vi "信号光谱3-拟合优化版本.vi"() -> ()   [LabVIEW 2018]
uses:
  <vilib>/Utility/file.llb/Write Delimited Spreadsheet (DBL).vi
  <vilib>/Analysis/NI_AALBase.lvlib
  <vilib>/ptbypt/NI_PtbyPt.lvlib
panel:
  in  "格式字符串":string
  in  "分隔符(Tab)":string
  in  "端口":u16
  in  "地址":string
  out "正在测量":bool
  in  "滤波阈值":dbl=1500.0 format="%#_13g"
  out "best fit":dbl[][](graph) caption="最佳拟合"
  out "范围内？":bool[](array[boolean])
  out "w":dbl
  out "xc":dbl
  out "拟合参数":dbl[](array[numeric])
  out "最终存储路径":path
  in  "停止程序":bool
  in  "上升下降沿/s":dbl format="%.2p"
  in  "延时/s":dbl format="%.2p"
  in  "占空比/%":dbl=3.0 format="%.2p"
  in  "高电平/V":dbl=4.0 format="%.2p"
  in  "频率/Hz":dbl=100.0 format="%.3p"
  in  "低电平/V":dbl min=0.0 max=5.0 format="%.2p"
  out "configure error out":errorcluster
  in  "设置参数":bool
  out "output control error  4":errorcluster
  in  "低电平持续输出":bool
  in  "Output 1":bool
  out "output control error  5":errorcluster
  in  "脉冲作用时间/s":dbl=1.0
  in  "测量高电平/V":dbl=4.0
  out "output control error  2":errorcluster
  in  "测量次数":i32=1
  in  "开始测量":bool
  in  "上升下降沿":i32(ring)=1 items=["上升沿", "下降沿"]
  in  "channel输出口":i32(ring) items=["Channel 1", "Channel 2"]
  in  "输出信号波形":u16(ring) items=["Pulse"]
  out "output control error  3":errorcluster
  out "Output":bool
  in  "VISA 信号发生器":refnum<visa-resource-name>="USB0::0x1AB1::0x0641::DG4E192200870::INSTR"
  out "Spectrum":cluster{"Y":dbl[], "Y":dbl[]}[](graph)
  in  "计数器":dbl=720.0
  out "波长范围":dbl[](array[numeric])
  in  "选项卡控件":enum32{"IHR 550", "CCD"}(tab)
  in  "Move To\nTarget Positions":bool
  out "Current UniqueID":string="Mono4"
  in  "Mono ID":string(combo)="Mono1"
  in  "Connect":bool
  out "Initialized JY":bool=TRUE
  in  "Force\nInitialization":bool
  in  "Target Grating":string(combo)="2"
  out "Current Description":string="1" caption="Description"
  out "Grating Index":i32=1
  out "Current Grating":dbl=1200.0
  out "Units":string="nm"
  out "Current WL":dbl=897.9988
  out "Exit Mirror\nPosition":i32(ring)=2 items=["EntranceMirror", "ExitMirror", "Front", "Side"]
  out "Entrance Mirror\nPosition":i32(ring)=2 items=["EntranceMirror", "ExitMirror", "Front", "Side"]
  out "Units 2":string="mm"
  out "Front Entrance":dbl
  in  "Target WL":dbl=2670.0
  in  "Exit Mirror":u16(ring)=3 caption="Target Position Exit Mirror" items=["Front"=2, "Side"=3]
  in  "Entrance Mirror":u16(ring)=2 caption="Target Position\nEntrance Mirror" items=["Front"=2, "Side"=3]
  in  "Target\nFront Entrance":dbl=1.0
  in  "Commande tab":T1(tab)
  in  "Area Number to Display":i32
  in  "Reformat":bool
  in  "GAIN":u16(ring)=2 caption="Device Name" items=["High Light", "Best Dynamic Range", "High Sensitivity"]
  in  "ADC":u16(ring) caption="Device Name" items=["20 kHz       ", " 1 MHz       ", " 1 MHz Ultra "]
  in  "Number of Areas :":u16=1 min=1 step=1
  in  "Integration time (ms) :":i16=5000
  out "Uniques ID":u16(ring) items=["CCD1", "CCD2"]
  in  "Device Name":u16(ring) items=["Synapse CCD (Lateral)", "Synapse_IGA (Axial)"]
  in  "Signal type :":enum16{"TTL Rising Edge", "TTL Falling Edge"}(ring)=enum."TTL Falling Edge"
  in  "Trigger Type :":u16(ring) items=["On Start"=1, "Per Acquisition"=2]
  in  "trigSigTypeString":string
  in  "trigEventString":string
  in  "Enable InputTriggers :":bool
  in  "Number of Cleans":i32=1
  in  "MultiAcqShutterMode":i32(ring)=3 items=["Open For All Spectra"=1, "Open for Each Spectrum"=3]
  in  "Accumulations:":u16=10 min=1 step=1
  in  "Multi Accumulation mode:":bool
  out "Y Pixels:":i32=256
  out "DataSize":i32=1024
  out "X Pixels:":i32=1024
  out "Firmware\nVersion":string="V1.20 CCD_4000"
  out "initialized ?":bool=TRUE
  in  "Continuous":bool
  in  "CCD Busy":bool
  out "indicator":string="Ready !"
  in  "initialize":bool
  in  "ShutterOpen":bool=TRUE caption="Shutter enable"
  in  "Acquire":bool
  in  "Temperature":bool
  in  "Setup":bool
  in  "起始波长":dbl=2406.79
  in  "终止波长":dbl=2919.91
  out "Acq Time(ms)":u32=3401
  in  "Save Backlight":bool
  in  "cut backlight":bool
  out "backlight":bool=TRUE
  in  "Close":bool=TRUE
  out "JYCCDLib.IJYCCDReqd":refnum<k7>
  out "areas :":i32[][](array[numeric])=[[1], [1], [1], [1024], [256], [1], [256]]
  in  "Constante de condition\n(Voir l'aide contextuelle)":bool
  out "temp graph":dbl(graph)=-134.538067
  out "ADC Number":i32[](array[numeric])=[0, 1, 2, 3, 4]
  out "Gain Number":i32[](array[numeric])=[10, 11, 12, 13, 8, 2]
  out "trigAddress":i32
  out "Data":i32[][](graph)
  out "error out":errorcluster
  out "Gratings":dbl[](array[numeric])=[1200.0, 300.0]
  out "Backlight":i32[][](graph)
  out "data 2":i32[][](graph)
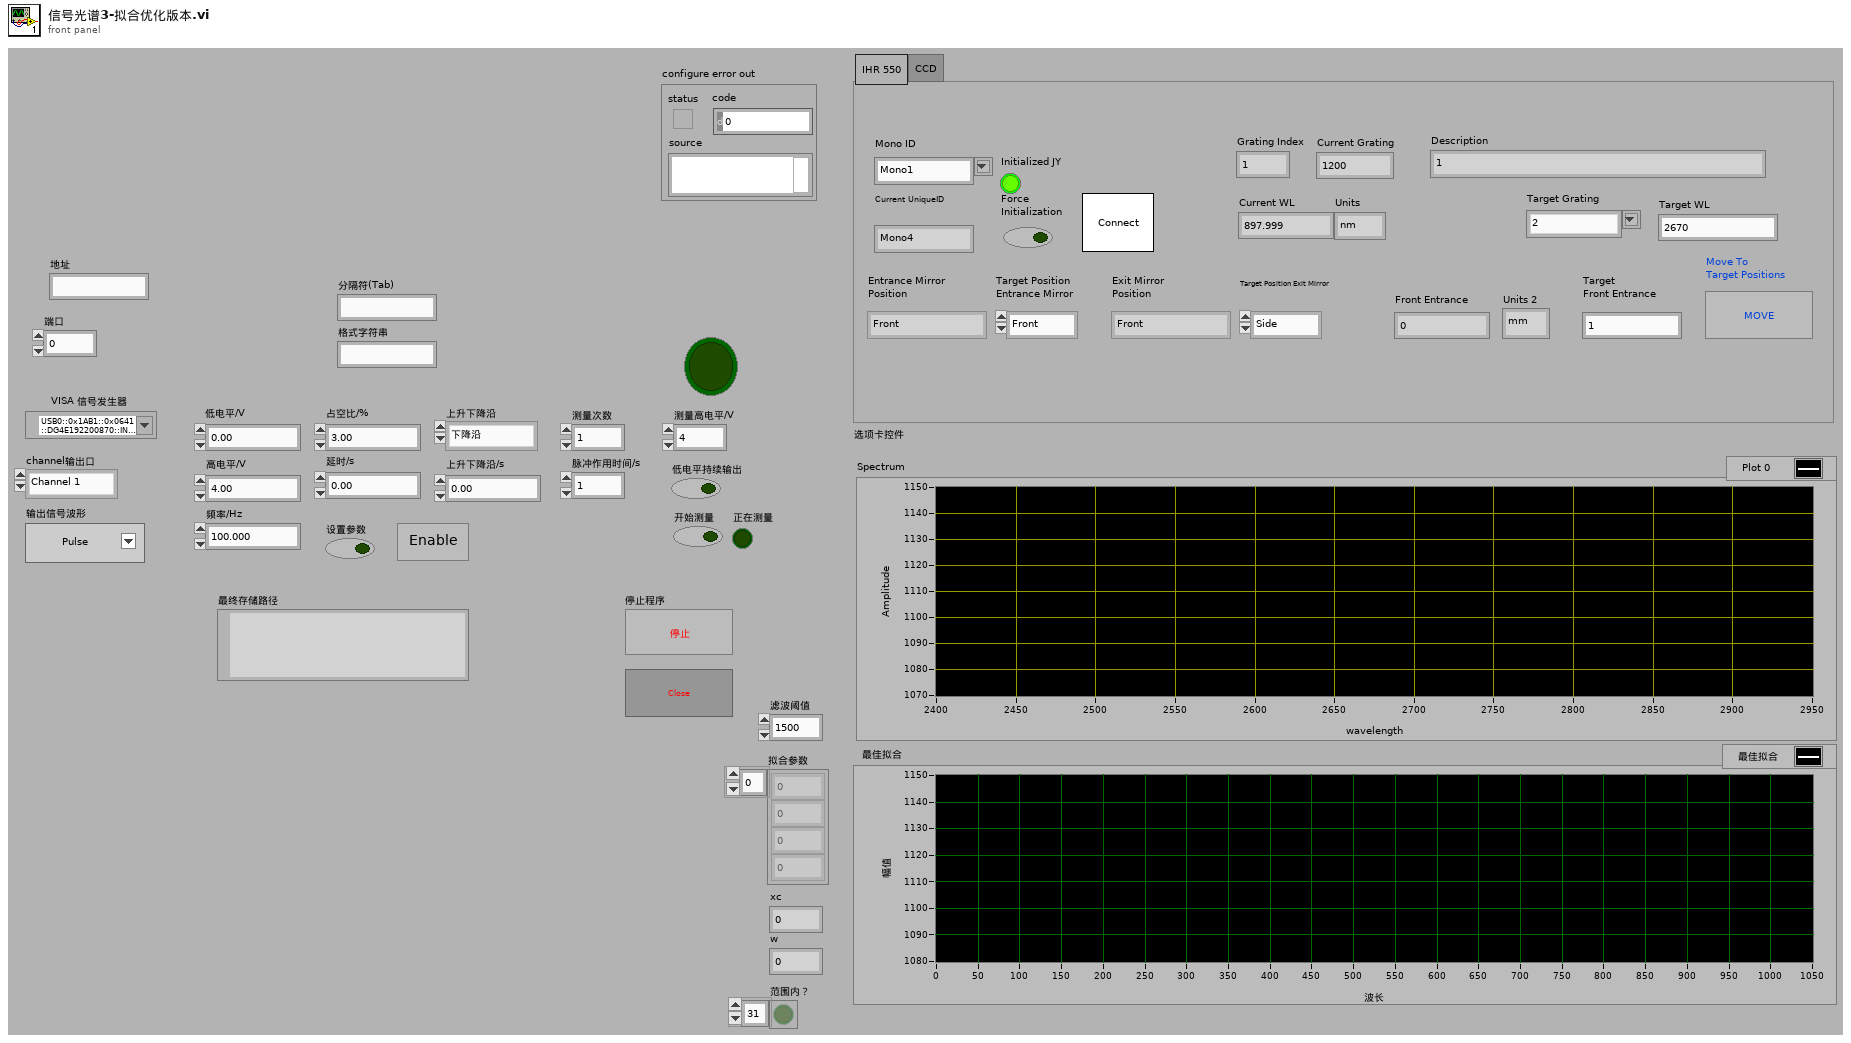
[diagram p1: front panel]
types:
  T1 = enum32{"Settings", "Trigger In", "Multi-Accu.", "Infos"}
  T2 = enum8{"Enabled", "Disabled", "Disabled and Grayed Out"}
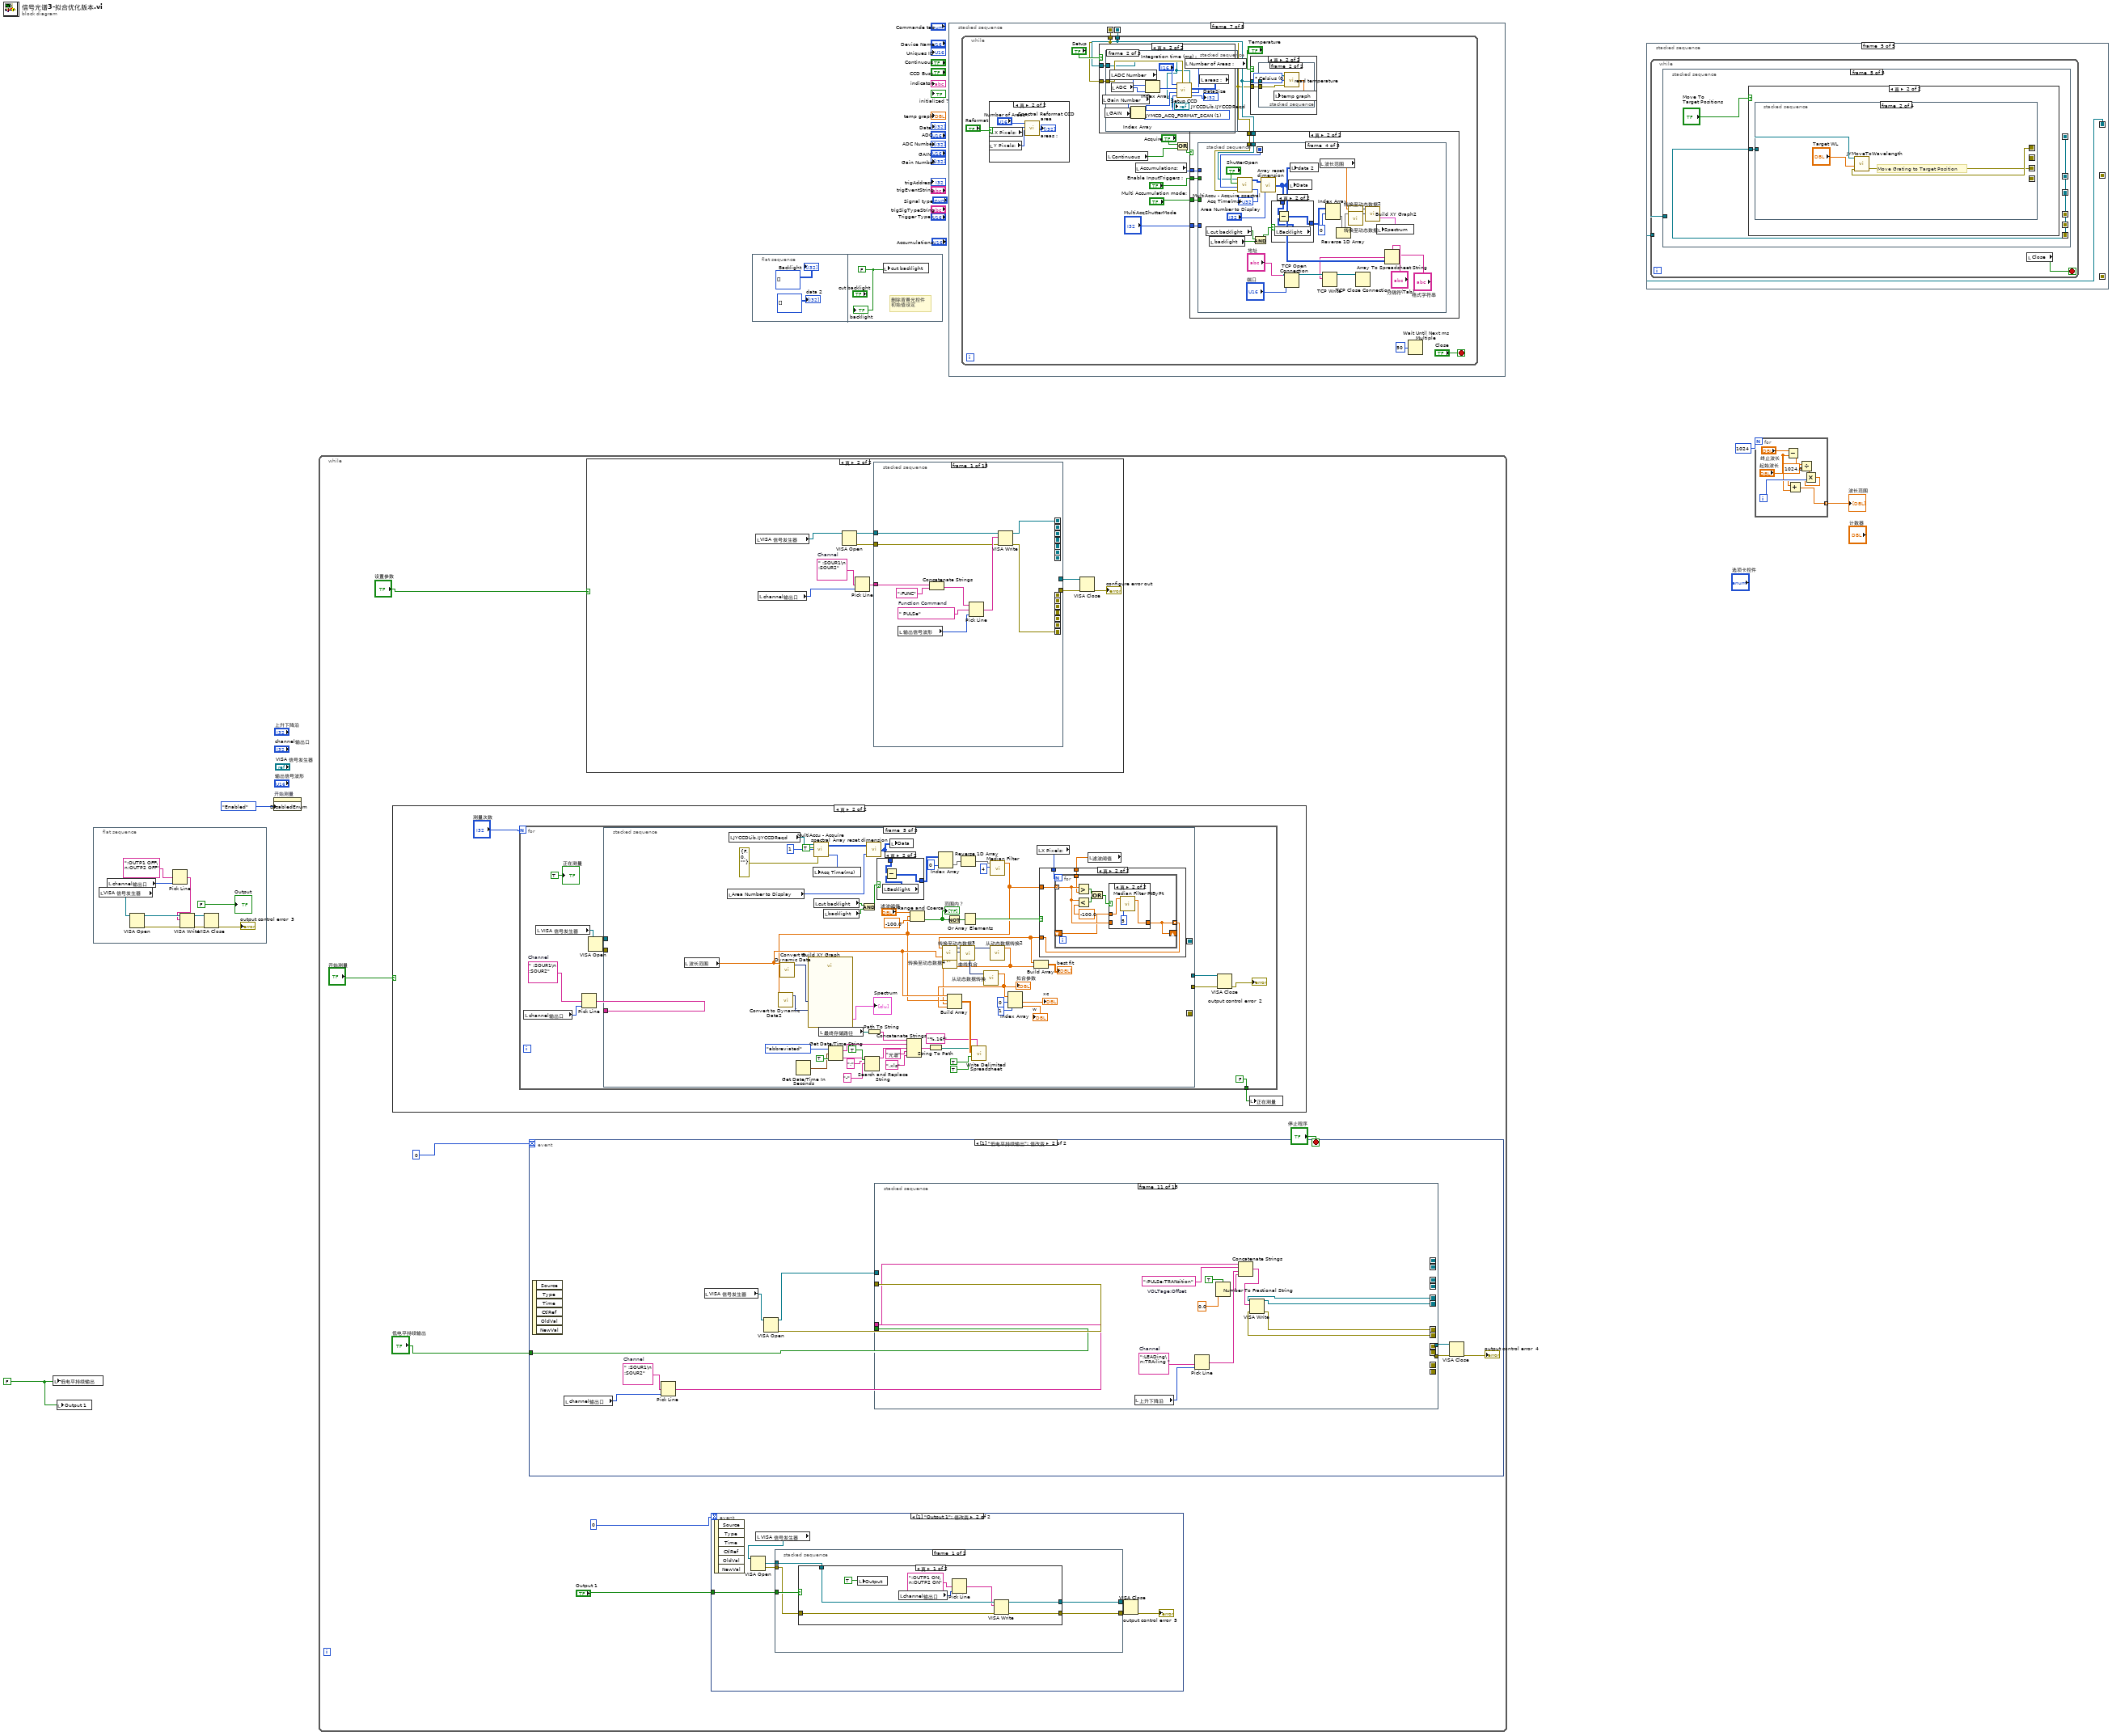
[diagram p0: block diagram]
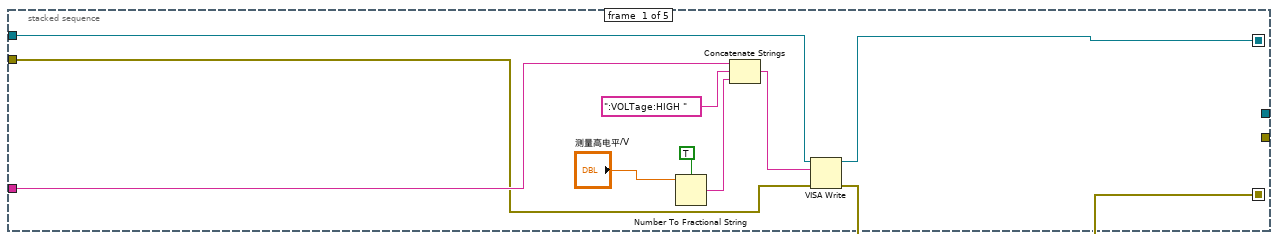
[diagram p3: hidden frame]
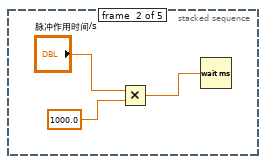
[diagram p4: hidden frame]
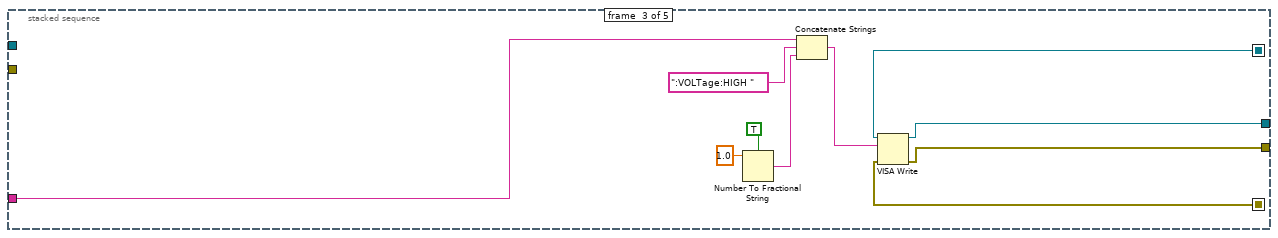
[diagram p5: hidden frame]
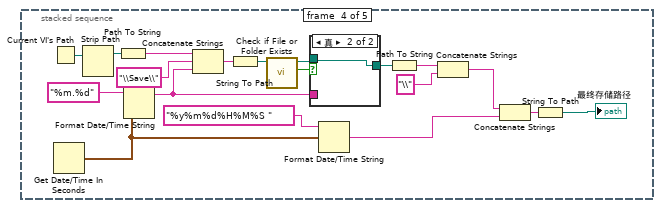
[diagram p6: hidden frame]
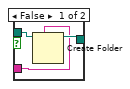
[diagram p7: hidden frame]
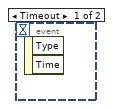
[diagram p11: hidden frame]
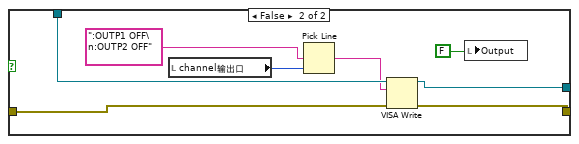
[diagram p12: hidden frame]
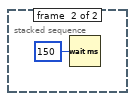
[diagram p13: hidden frame]
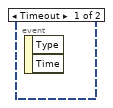
[diagram p14: hidden frame]
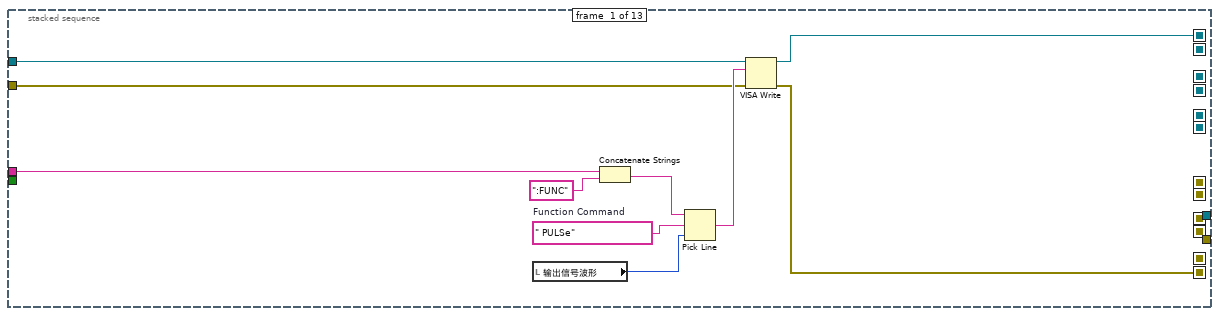
[diagram p15: hidden frame]
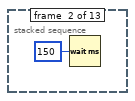
[diagram p16: hidden frame]
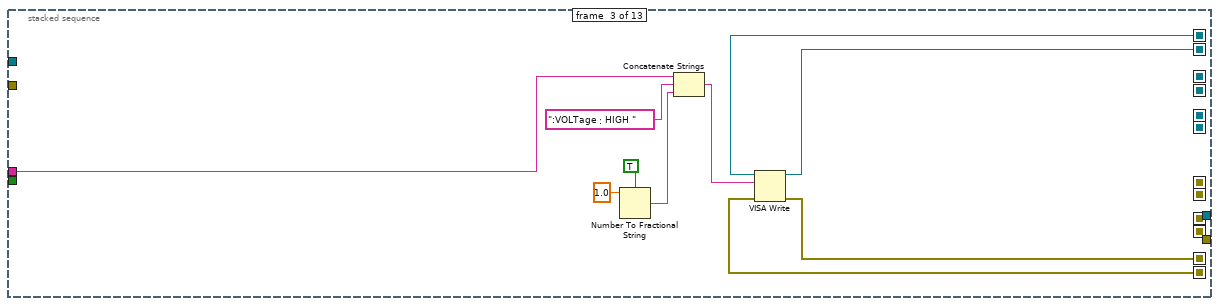
[diagram p17: hidden frame]
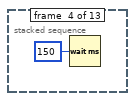
[diagram p18: hidden frame]
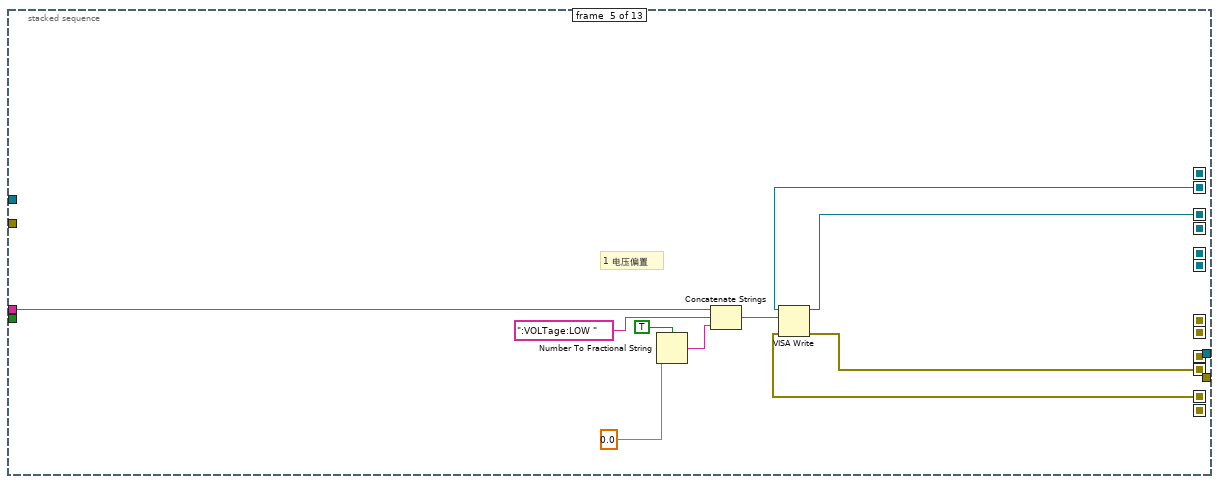
[diagram p19: hidden frame]
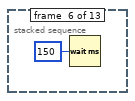
[diagram p20: hidden frame]
diagram:
  w1 = FALSE
  n1 = local write "低电平持续输出"(w1) -> ()
  n2 = local write "Output 1"(w1) -> ()
  n3 = flat-sequence {
    frame #0 {
      n4 = local read "VISA 信号发生器"() -> (w8:refnum<visa-resource-name>)
      n5 = local read "channel输出口"() -> (w6:i32)
      n6 = VISA Open(VISA resource name=w8) -> (VISA resource name=w14:refnum<visa-resource-name>, error out=w13:errorcluster)  [unwired: 4 in]
      n7 = Pick Line(multi-line string=":OUTP1 OFF\n:OUTP2 OFF" ("write buffer"), line index=w6) -> (output string=w5:string)  [unwired: 1 in]
      n8 = VISA Write(VISA resource name=w14, write buffer=w5, error in (no error)=w13) -> (VISA resource name out=w11:refnum<visa-resource-name>, error out=w10:errorcluster)  [unwired: 1 out]
      n9 = VISA Close(VISA resource name=w11, error in (no error)=w10) -> (error out=→"output control error  3":errorcluster)
      "Output" <- FALSE ("布尔")
    }
  }
  n10 = property on="开始测量" class="Bool"("DisabledEnum"=T2."Enabled" ("禁用")) -> ()  [unwired: 2 in, 2 out]
  n11 = while {
    stop <- "停止程序" stop-if-true
    n12 = case shown="真" "开始测量" {
      frame False {
      }
      frame True {
        n13 = for {
          N: "测量次数" -> [_]
          tunnel: [FALSE] -> w22
          w27 = " :SOUR1\n :SOUR2"  # Channel
          n14 = local read "channel输出口"() -> (w28:i32)
          n15 = local read "VISA 信号发生器"() -> (w34:refnum<visa-resource-name>)
          n16 = Pick Line(multi-line string=w27, line index=w28) -> (output string=w26:string)  [unwired: 1 in]
          n17 = VISA Open(VISA resource name=w34) -> (VISA resource name=w33:refnum<visa-resource-name>, error out=w32:errorcluster)  [unwired: 4 in]
          n18 = stacked-sequence {
            seq-local: [w37 _ _ _ _] -> [_ _ w50 _ _]
            seq-local: [w36 _ _ _ _] -> [_ _ w49 _ _]
            tunnel: w33 -> [w39 _ _ _ _]
            tunnel: w32 -> [w38 _ _ _ _]
            tunnel: [_ _ w52 _ _] -> w31
            tunnel: [_ _ w51 _ _] -> w30
            tunnel: w26 -> [w40 _ w48 _ _]
            frame #0 {
              n19 = Number To Fractional String(use system decimal point (T)=TRUE ("使用系统小数点(T)"), number="测量高电平/V") -> (F-format string=w42:string)  [unwired: 2 in]
              n20 = Concatenate Strings ("连接字符串")(w40, ":VOLTage:HIGH ", w42) -> (w41:string)
              n21 = VISA Write(VISA resource name=w39, write buffer=w41, error in (no error)=w38) -> (VISA resource name out=w37:refnum<visa-resource-name>, error out=w36:errorcluster)  [unwired: 1 out]
            }
            frame #1 {
              n22 = Multiply(x="脉冲作用时间/s", y=1000.0) -> (x*y=w45:dbl)
              n23 = Wait (ms)(milliseconds to wait=w45) -> ()  [unwired: 1 out]
            }
            frame #2 {
              n24 = Number To Fractional String(use system decimal point (T)=TRUE ("使用系统小数点(T)"), number=1.0 ("数字")) -> (F-format string=w55:string)  [unwired: 2 in]
              n25 = Concatenate Strings ("连接字符串")(w48, ":VOLTage:HIGH ", w55) -> (w54:string)
              n26 = VISA Write(VISA resource name=w50, write buffer=w54, error in (no error)=w49) -> (VISA resource name out=w52:refnum<visa-resource-name>, error out=w51:errorcluster)  [unwired: 1 out]
            }
            frame #3 {
              n27 = Current VI's Path() -> (path=w63:path)
              n28 = Get Date/Time In Seconds() -> (seconds since 1Jan1904=w65:timestamp)
              n29 = Strip Path(path=w63) -> (stripped path=w64:path)  [unwired: 1 out]
              n30 = Path To String(path=w64) -> (string=w66:string)
              n31 = Format Date/Time String(time format string (%c)="%m.%d" ("时间格式字符串(%c)"), seconds (now)=w65) -> (date/time string=w72:string)  [unwired: 1 in]
              n32 = Concatenate Strings(w66, "\\Save\\" ("字符串"), w72) -> (w67:string)
              n33 = String To Path(string=w67) -> (path=w68:path)
              n34 = call <vilib>:"Check if File or Folder Exists.vi"("path"=w68) -> ("file or folder exists?"=w69:bool, "dup path"=w71:path)  [unwired: 8 in, 1 out]
              n35 = case shown="真" w69 {
                tunnel: [w79 w80] -> w70
                tunnel: w71 -> [w78 w80]
                tunnel: w72 -> [w77 _]
                frame False {
                  n36 = Create Folder(prompt (Create Folder)=w77, path (use dialog)=w78) -> (created path=w79:path)  [unwired: 1 in, 2 out]
                }
                frame True {
                }
              }
              n37 = Format Date/Time String(time format string (%c)="%y%m%d%H%M%S " ("时间格式字符串(%c)"), seconds (now)=w65) -> (date/time string=w75:string)  [unwired: 1 in]
              n38 = Path To String(path=w70) -> (string=w73:string)
              n39 = Concatenate Strings(w73, "\\" ("字符串")) -> (w74:string)
              n40 = Concatenate Strings(w74, w75) -> (w62:string)
              n41 = String To Path(string=w62) -> (path=→"最终存储路径":path)
            }
            frame #4 {
              n42 = local read "波长范围"() -> (w103:dbl[])
              n43 = local read "Area Number to Display"() -> (w113:i32)
              n44 = local read "JYCCDLib.IJYCCDReqd"() -> (w109:refnum<k7>)
              n45 = call "Convert to Dynamic Data"("Array"=w103) -> ("Dynamic Data Type"=w106:dynamicdata)  [unwired: 3 in]
              n46 = Get Date/Time In Seconds() -> (seconds since 1Jan1904=w122:timestamp)
              n47 = call "MultiAccu - Acquire spectral.vi"("error in"=errorcluster {"status"=FALSE, "code"=0, "source"=""}, "Accumulations:"=u16 1, "ShutterOpen"=TRUE, "JYCCDLib.IJYCCDReqd"=w109) -> ("Acq Time(ms)"=w115:u32, "Array Out"=w114:i32[][][])  [unwired: 1 out]
              n48 = local write "Acq Time(ms)"(w115) -> ()
              n49 = local read "cut backlight"() -> (w94:bool)
              n50 = local read "最终存储路径"() -> (w136:path)
              n51 = local read "backlight"() -> (w92:bool)
              n52 = Get Date/Time String(date format (0)=enum16{"short", "long", "abbreviated"}."abbreviated" ("日期格式(0)"), seconds (now)=w122, want seconds? (F)=TRUE ("需要秒？(F)")) -> (date string=w130:string, time string=w125:string)
              n53 = And(x=w94, y=w92) -> (x .and. y?=w93:bool)
              n54 = Search and Replace String(replace all?=TRUE ("替换全部？(F)"), input string=w125, search string=":" ("搜索字符串"), replace string="-" ("替换字符串(\"\")")) -> (result string=w129:string)  [unwired: 4 in, 3 out]
              n55 = call "Array reset dimension.vi"("Area Number"=w113, "Array In"=w114) -> ("Array Out"=w96:i32[][])
              n56 = Path To String(path=w136) -> (string=w119:string)
              n57 = case shown="真" w93 {
                tunnel: [w157 w159] -> w95
                tunnel: w96 -> [w157 w158]
                frame False {
                }
                frame True {
                  n58 = local read "Backlight"() -> (w160:i32[][])
                  n59 = Subtract(x=w158, y=w160) -> (x-y=w159:i32[][])
                }
              }
              n60 = local write "Data"(w96) -> ()
              n61 = Concatenate Strings(w119, w130, w129, "光谱" ("字符串"), ".xls" ("字符串")) -> (w134:string)
              n62 = String To Path(string=w134) -> (path=w135:path)
              n63 = Index Array(array=w95, index (row)=0 ("索引 (行)")) -> (element=w137:i32[])  [unwired: 1 in]
              n64 = call "转换至动态数据4"("Array"=w103) -> ("Dynamic Data Type"=w102:dynamicdata)  [unwired: 3 in]
              n65 = Reverse 1D Array(array=w137) -> (reversed array=w138:i32[])
              n66 = call <vilib>:"Median Filter.vi"("left rank"=4, "X"=w138) -> ("Filtered X"=w87:dbl[])  [unwired: 8 in, 1 out]
              n67 = call "Convert to Dynamic Data2"("Array"=w87) -> ("Dynamic Data Type"=w105:dynamicdata)  [unwired: 3 in]
              n68 = call "Build XY Graph"("Y Input"=w105, "X Input"=w106) -> ("XY Graph"=→"Spectrum":cluster{"Y":dbl[], "Y":dbl[]}[])  [unwired: 8 in, 1 out]
              n69 = In Range and Coerce(upper limit="滤波阈值", x=w87, lower limit=-100.0) -> (In Range?=w86:bool[])  [unwired: 1 out]
              "范围内？" <- w86
              n70 = Not(x=w86) -> (.not. x?=w85:bool[])
              n71 = Or Array Elements(Boolean array=w85) -> (logical OR=w89:bool)
              n72 = local read "X Pixels:"() -> (w88:i32)
              n73 = local read "滤波阈值"() -> (w81:dbl)
              n74 = case shown="真" w89 {
                tunnel: w88 -> [_ w144]
                tunnel: w87 -> [w140 w143]
                tunnel: [w140 w142] -> w84
                tunnel: w81 -> [_ w141]
                frame False {
                }
                frame True {
                  n75 = for {
                    N: w144 -> [_]
                    tunnel: w143 -> [w148] mode=indexing
                    tunnel: [w147] -> w142 mode=indexing
                    shift-right: [w147] -> _
                    shift-left: _ -> [w146]
                    tunnel: w141 -> [w145]
                    n76 = Greater?(x=w148, y=w145) -> (0:w150:bool)
                    n77 = Less?(x=w148, y=-100.0) -> (x < y?=w151:bool)
                    n78 = Or(x=w150, y=w151) -> (x .or. y?=w149:bool)
                    n79 = case shown="真" w149 {
                      tunnel: w148 -> [w153 _]
                      tunnel: [w153 w155] -> w147
                      tunnel: w146 -> [_ w156]
                      frame False {
                      }
                      frame True {
                        n80 = call <vilib>:"Median Filter PtByPt.vi"("rank"=5, "x"=w156) -> ("Filtered x"=w155:dbl)  [unwired: 2 in, 1 out]
                      }
                    }
                  }
                }
              }
              n81 = call "转换至动态数据3"("Array"=w84) -> ("Dynamic Data Type"=w104:dynamicdata)  [unwired: 3 in]
              n82 = call "曲线拟合"("Locations"=w102, "Signals"=w104) -> ("best fit"=w108:dynamicdata, "non-linear coefficients"=w107:dynamicdata)  [unwired: 5 in, 3 out]
              n83 = call "从动态数据转换"("Dynamic Data Type"=w107) -> ("Array"=w99:dbl[])  [unwired: 3 in]
              "拟合参数" <- w99
              n84 = call "从动态数据转换2"("Dynamic Data Type"=w108) -> ("Array"=w83:dbl[])  [unwired: 3 in]
              n85 = Build Array(w103, w87, w83, w99) -> (w139:dbl[][])
              n86 = call-poly <vilib>:"Write Delimited Spreadsheet.vi"("file path (dialog if empty)"=w135, "format (%.3f)"="%.16f", "2D data"=w139, "append to file? (new file:F)"=TRUE ("append to file? (F)"), "transpose? (no:F)"=TRUE ("transpose? (F)")) -> ()  [unwired: 9 in, 2 out]
              n87 = Index Array(array=w99, index #1=0 ("索引"), index #2=1 ("索引")) -> (element #1=→"xc":dbl, element #2=→"w":dbl)
              n88 = Build Array(w84, w83) -> (→"best fit":dbl[][])
            }
          }
          n89 = VISA Close(VISA resource name=w31, error in (no error)=w30) -> (error out=→"output control error  2":errorcluster)
          "正在测量" <- TRUE
        }
        n90 = local write "正在测量"(w22) -> ()
      }
    }
    n91 = event shown="[1] \"低电平持续输出\": 值改变" {
      selector: _ -> [_ _]
      dyn-events: _ -> [_ _]
      timeout: u32 0 ("Time") -> [_ _]
      tunnel: "低电平持续输出" -> [_ w190]
      event Timeout {
        n92 = event-data() -> ()  [unwired: 1 in, 2 out]
      }
      event "低电平持续输出": Value Change {
        w194 = " :SOUR1\n :SOUR2"  # Channel
        n93 = event-data() -> ()  [unwired: 1 in, 6 out]
        n94 = local read "channel输出口"() -> (w195:i32)
        n95 = Pick Line(multi-line string=w194, line index=w195) -> (output string=w193:string)  [unwired: 1 in]
        n96 = local read "VISA 信号发生器"() -> (w198:refnum<visa-resource-name>)
        n97 = VISA Open(VISA resource name=w198) -> (VISA resource name=w197:refnum<visa-resource-name>, error out=w196:errorcluster)  [unwired: 4 in]
        n98 = stacked-sequence {
          seq-local: [w204 _ _ _ _ _ _ _ _ _ _ _ _] -> [_ _ w219 _ _ _ _ _ _ _ _ _ _]
          seq-local: [w203 _ _ _ _ _ _ _ _ _ _ _ _] -> [_ _ w218 _ _ _ _ _ _ _ _ _ _]
          seq-local: [_ _ w217 _ _ _ _ _ _ _ _ _ _] -> [_ _ _ _ w222 _ _ _ _ _ _ _ _]
          seq-local: [_ _ w216 _ _ _ _ _ _ _ _ _ _] -> [_ _ _ _ w223 _ _ _ _ _ _ _ _]
          seq-local: [_ _ _ _ w231 _ _ _ _ _ _ _ _] -> [_ _ _ _ _ _ w242 _ _ _ _ _ _]
          seq-local: [_ _ _ _ w230 _ _ _ _ _ _ _ _] -> [_ _ _ _ _ _ w241 _ _ _ _ _ _]
          seq-local: [_ _ _ _ _ _ w235 _ _ _ _ _ _] -> [_ _ _ _ _ _ _ _ w245 _ _ _ _]
          seq-local: [_ _ _ _ _ _ w234 _ _ _ _ _ _] -> [_ _ _ _ _ _ _ _ w244 _ _ _ _]
          seq-local: [_ _ _ _ _ _ _ _ w248 _ _ _ _] -> [_ _ _ _ _ _ _ _ _ _ w259 _ _]
          seq-local: [_ _ _ _ _ _ _ _ w247 _ _ _ _] -> [_ _ _ _ _ _ _ _ _ _ w258 _ _]
          seq-local: [_ _ _ _ _ _ _ _ _ _ w256 _ _] -> [_ _ _ _ _ _ _ _ _ _ _ _ w273]
          seq-local: [_ _ _ _ _ _ _ _ _ _ w255 _ _] -> [_ _ _ _ _ _ _ _ _ _ _ _ w272]
          tunnel: w197 -> [w209 _ _ _ _ _ _ _ _ _ _ _ _]
          tunnel: w196 -> [w202 _ _ _ _ _ _ _ _ _ _ _ _]
          tunnel: w193 -> [w201 _ w215 _ w228 _ w239 _ w249 _ w262 _ _]
          tunnel: [_ _ _ _ _ _ _ _ _ _ _ _ w271] -> w192
          tunnel: [_ _ _ _ _ _ _ _ _ _ _ _ w269] -> w191
          tunnel: w190 -> [_ _ _ _ _ _ _ _ _ _ _ _ w270]
          frame #0 {
            w206 = " PULSe"  # Function Command
            n99 = local read "输出信号波形"() -> (w200:u16)
            n100 = Concatenate Strings(w201, ":FUNC" ("string (\"\")")) -> (w207:string)
            n101 = Pick Line(string ("")=w207, multi-line string=w206, line index=w200) -> (output string=w205:string)
            n102 = VISA Write(VISA resource name=w209, write buffer=w205, error in (no error)=w202) -> (VISA resource name out=w204:refnum<visa-resource-name>, error out=w203:errorcluster)  [unwired: 1 out]
          }
          frame #1 {
            n103 = Wait (ms)(milliseconds to wait=u32 150) -> ()  [unwired: 1 out]
          }
          frame #2 {
            n104 = Number To Fractional String(use system decimal point (T)=TRUE ("使用系统小数点(T)"), number=1.0 ("数字")) -> (F-format string=w213:string)  [unwired: 2 in]
            n105 = Concatenate Strings ("连接字符串")(w215, ":VOLTage：HIGH ", w213) -> (w212:string)
            n106 = VISA Write(VISA resource name=w219, write buffer=w212, error in (no error)=w218) -> (VISA resource name out=w217:refnum<visa-resource-name>, error out=w216:errorcluster)  [unwired: 1 out]
          }
          frame #3 {
            n107 = Wait (ms)(milliseconds to wait=u32 150) -> ()  [unwired: 1 out]
          }
          frame #4 {
            # "1 电压偏置"
            n108 = Number To Fractional String(use system decimal point (T)=TRUE ("使用系统小数点(T)"), number=0.0 ("数字")) -> (F-format string=w226:string)  [unwired: 2 in]
            n109 = Concatenate Strings(w228, ":VOLTage:LOW ", w226) -> (w227:string)
            n110 = VISA Write(VISA resource name=w222, write buffer=w227, error in (no error)=w223) -> (VISA resource name out=w231:refnum<visa-resource-name>, error out=w230:errorcluster)  [unwired: 1 out]
          }
          frame #5 {
            n111 = Wait (ms)(milliseconds to wait=u32 150) -> ()  [unwired: 1 out]
          }
          frame #6 {
            n112 = local read "channel输出口"() -> (w237:i32)
            n113 = Pick Line(multi-line string=":OUTP1:IMPedance \n:OUTP2:IMPedance " ("write buffer"), line index=w237) -> (output string=w236:string)  [unwired: 1 in]
            n114 = Concatenate Strings ("连接字符串")(w239, w236, "INFINITY") -> (w240:string)
            n115 = VISA Write(VISA resource name=w242, write buffer=w240, error in (no error)=w241) -> (VISA resource name out=w235:refnum<visa-resource-name>, error out=w234:errorcluster)  [unwired: 1 out]
          }
          frame #7 {
            n116 = Wait (ms)(milliseconds to wait=u32 150) -> ()  [unwired: 1 out]
          }
          frame #8 {
            n117 = Number To Fractional String(use system decimal point (T)=TRUE ("使用系统小数点(T)"), number=0.0 ("数字")) -> (F-format string=w252:string)  [unwired: 2 in]
            n118 = Concatenate Strings(w249, ":PULSe:DELay ", w252) -> (w250:string)
            n119 = VISA Write(VISA resource name=w245, write buffer=w250, error in (no error)=w244) -> (VISA resource name out=w248:refnum<visa-resource-name>, error out=w247:errorcluster)  [unwired: 1 out]
          }
          frame #9 {
            n120 = Wait (ms)(milliseconds to wait=u32 150) -> ()  [unwired: 1 out]
          }
          frame #10 {
            w263 = ":LEADing\n:TRAiling "  # Channel
            w267 = ":PULSe:TRANsition"  # VOLTage:Offset
            n121 = local read "上升下降沿"() -> (w264:i32)
            n122 = Pick Line(multi-line string=w263, line index=w264) -> (output string=w260:string)  [unwired: 1 in]
            n123 = Number To Fractional String(use system decimal point (T)=TRUE ("使用系统小数点(T)"), number=0.0 ("数字")) -> (F-format string=w261:string)  [unwired: 2 in]
            n124 = Concatenate Strings(w262, w267, w260, w261) -> (w265:string)
            n125 = VISA Write(VISA resource name=w259, write buffer=w265, error in (no error)=w258) -> (VISA resource name out=w256:refnum<visa-resource-name>, error out=w255:errorcluster)  [unwired: 1 out]
          }
          frame #11 {
            n126 = Wait (ms)(milliseconds to wait=u32 150) -> ()  [unwired: 1 out]
          }
          frame #12 {
            n127 = case shown="假" w270 {
              tunnel: w273 -> [w281 w282]
              tunnel: [w280 w289] -> w269
              tunnel: w272 -> [w279 w287]
              tunnel: [w278 w288] -> w271
              frame True {
                n128 = local write "Output"(TRUE ("布尔")) -> ()
                n129 = local read "channel输出口"() -> (w275:i32)
                n130 = Pick Line(multi-line string=":OUTP1 ON\n:OUTP2 ON" ("write buffer"), line index=w275) -> (output string=w274:string)  [unwired: 1 in]
                n131 = VISA Write(VISA resource name=w281, write buffer=w274, error in (no error)=w279) -> (VISA resource name out=w278:refnum<visa-resource-name>, error out=w280:errorcluster)  [unwired: 1 out]
              }
              frame False {
                n132 = local read "channel输出口"() -> (w284:i32)
                n133 = Pick Line(multi-line string=":OUTP1 OFF\n:OUTP2 OFF" ("write buffer"), line index=w284) -> (output string=w283:string)  [unwired: 1 in]
                n134 = VISA Write(VISA resource name=w282, write buffer=w283, error in (no error)=w287) -> (VISA resource name out=w288:refnum<visa-resource-name>, error out=w289:errorcluster)  [unwired: 1 out]
                n135 = local write "Output"(FALSE ("布尔")) -> ()
              }
            }
          }
        }
        n136 = VISA Close(VISA resource name=w192, error in (no error)=w191) -> (error out=→"output control error  4":errorcluster)
      }
    }
    n137 = case shown="真" "设置参数" {
      frame False {
      }
      frame True {
        w295 = " :SOUR1\n :SOUR2"  # Channel
        n138 = local read "VISA 信号发生器"() -> (w291:refnum<visa-resource-name>)
        n139 = local read "channel输出口"() -> (w290:i32)
        n140 = VISA Open(VISA resource name=w291) -> (VISA resource name=w297:refnum<visa-resource-name>, error out=w298:errorcluster)  [unwired: 4 in]
        n141 = Pick Line(multi-line string=w295, line index=w290) -> (output string=w294:string)  [unwired: 1 in]
        n142 = stacked-sequence {
          seq-local: [w303 _ _ _ _ _ _ _ _ _ _ _ _ _ _] -> [_ _ w318 _ _ _ _ _ _ _ _ _ _ _ _]
          seq-local: [w302 _ _ _ _ _ _ _ _ _ _ _ _ _ _] -> [_ _ w317 _ _ _ _ _ _ _ w356 _ _ _ _]
          seq-local: [_ _ w316 _ _ _ _ _ _ _ _ _ _ _ _] -> [_ _ _ _ w327 _ _ _ _ _ _ _ _ _ _]
          seq-local: [_ _ w315 _ _ _ _ _ _ _ _ _ _ _ _] -> [_ _ _ _ w326 _ _ _ _ _ _ _ _ _ _]
          seq-local: [_ _ _ _ w325 _ _ _ _ _ _ _ _ _ _] -> [_ _ _ _ _ _ w333 _ _ _ _ _ _ _ _]
          seq-local: [_ _ _ _ w322 _ _ _ _ _ _ _ _ _ _] -> [_ _ _ _ _ _ w332 _ _ _ _ _ _ _ _]
          seq-local: [_ _ _ _ _ _ w340 _ _ _ _ _ _ _ _] -> [_ _ _ _ _ _ _ _ w351 _ _ _ _ _ _]
          seq-local: [_ _ _ _ _ _ w339 _ _ _ _ _ _ _ _] -> [_ _ _ _ _ _ _ _ w350 _ _ _ _ _ _]
          seq-local: [_ _ _ _ _ _ _ _ w344 _ _ _ _ _ _] -> [_ _ _ _ _ _ _ _ _ _ w357 _ _ _ _]
          seq-local: [_ _ _ _ _ _ _ _ w343 _ _ _ _ _ _] -> [_ _ _ _ _ _ _ _ _ _ _ _ _ _ _]
          seq-local: [_ _ _ _ _ _ _ _ _ _ w353 _ _ _ _] -> [_ _ _ _ _ _ _ _ _ _ _ _ w367 _ _]
          seq-local: [_ _ _ _ _ _ _ _ _ _ w354 _ _ _ _] -> [_ _ _ _ _ _ _ _ _ _ _ _ w366 _ _]
          seq-local: [_ _ _ _ _ _ _ _ _ _ _ _ w365 _ _] -> [_ _ _ _ _ _ _ _ _ _ _ _ _ _ w378]
          seq-local: [_ _ _ _ _ _ _ _ _ _ _ _ w364 _ _] -> [_ _ _ _ _ _ _ _ _ _ _ _ _ _ w377]
          tunnel: w297 -> [w308 _ _ _ _ _ _ _ _ _ _ _ _ _ _]
          tunnel: w298 -> [w301 _ _ _ _ _ _ _ _ _ _ _ _ _ _]
          tunnel: w294 -> [w300 _ w314 _ w321 _ w337 _ w348 _ w358 _ w368 _ w381]
          tunnel: [_ _ _ _ _ _ _ _ _ _ _ _ _ _ w376] -> w293
          tunnel: [_ _ _ _ _ _ _ _ _ _ _ _ _ _ w375] -> w292
          frame #0 {
            w305 = " PULSe"  # Function Command
            n143 = local read "输出信号波形"() -> (w299:u16)
            n144 = Concatenate Strings(w300, ":FUNC" ("string (\"\")")) -> (w306:string)
            n145 = Pick Line(string ("")=w306, multi-line string=w305, line index=w299) -> (output string=w304:string)
            n146 = VISA Write(VISA resource name=w308, write buffer=w304, error in (no error)=w301) -> (VISA resource name out=w303:refnum<visa-resource-name>, error out=w302:errorcluster)  [unwired: 1 out]
          }
          frame #1 {
            n147 = Wait (ms)(milliseconds to wait=u32 150) -> ()  [unwired: 1 out]
          }
          frame #2 {
            n148 = Number To Fractional String(use system decimal point (T)=TRUE ("使用系统小数点(T)"), number="低电平/V") -> (F-format string=w312:string)  [unwired: 2 in]
            n149 = Concatenate Strings ("连接字符串")(w314, ":VOLTage:LOW ", w312) -> (w311:string)
            n150 = VISA Write(VISA resource name=w318, write buffer=w311, error in (no error)=w317) -> (VISA resource name out=w316:refnum<visa-resource-name>, error out=w315:errorcluster)  [unwired: 1 out]
          }
          frame #3 {
            n151 = Wait (ms)(milliseconds to wait=u32 150) -> ()  [unwired: 1 out]
          }
          frame #4 {
            # "1 频率"
            n152 = Concatenate Strings(w321, ":FREQ ") -> (w328:string)
            n153 = Format Into String ("格式化写入字符串")(initial string=w328, "频率/Hz") -> (resulting string=w329:string)  [unwired: 2 in, 1 out]
            n154 = VISA Write(VISA resource name=w327, write buffer=w329, error in (no error)=w326) -> (VISA resource name out=w325:refnum<visa-resource-name>, error out=w322:errorcluster)  [unwired: 1 out]
          }
          frame #5 {
            n155 = Wait (ms)(milliseconds to wait=u32 150) -> ()  [unwired: 1 out]
          }
          frame #6 {
            n156 = Number To Fractional String(use system decimal point (T)=TRUE ("使用系统小数点(T)"), number="高电平/V") -> (F-format string=w334:string)  [unwired: 2 in]
            n157 = Concatenate Strings(w337, ":VOLTage:HIGH ", w334) -> (w336:string)
            n158 = VISA Write(VISA resource name=w333, write buffer=w336, error in (no error)=w332) -> (VISA resource name out=w340:refnum<visa-resource-name>, error out=w339:errorcluster)  [unwired: 1 out]
          }
          frame #7 {
            n159 = Wait (ms)(milliseconds to wait=u32 150) -> ()  [unwired: 1 out]
          }
          frame #8 {
            n160 = local read "channel输出口"() -> (w346:i32)
            n161 = Pick Line(multi-line string=":OUTP1:IMPedance \n:OUTP2:IMPedance " ("write buffer"), line index=w346) -> (output string=w345:string)  [unwired: 1 in]
            n162 = Concatenate Strings ("连接字符串")(w348, w345, "INFINITY") -> (w349:string)
            n163 = VISA Write(VISA resource name=w351, write buffer=w349, error in (no error)=w350) -> (VISA resource name out=w344:refnum<visa-resource-name>, error out=w343:errorcluster)  [unwired: 1 out]
          }
          frame #9 {
            n164 = Wait (ms)(milliseconds to wait=u32 150) -> ()  [unwired: 1 out]
          }
          frame #10 {
            n165 = Number To Fractional String(use system decimal point (T)=TRUE ("使用系统小数点(T)"), number="占空比/%") -> (F-format string=w360:string)  [unwired: 2 in]
            n166 = Concatenate Strings(w358, ":PULSe:DCYCle ", w360) -> (w355:string)
            n167 = VISA Write(VISA resource name=w357, write buffer=w355, error in (no error)=w356) -> (VISA resource name out=w353:refnum<visa-resource-name>, error out=w354:errorcluster)  [unwired: 1 out]
          }
          frame #11 {
            n168 = Wait (ms)(milliseconds to wait=u32 150) -> ()  [unwired: 1 out]
          }
          frame #12 {
            n169 = Number To Fractional String(use system decimal point (T)=TRUE ("使用系统小数点(T)"), number="延时/s") -> (F-format string=w371:string)  [unwired: 2 in]
            n170 = Concatenate Strings(w368, ":PULSe:DELay ", w371) -> (w369:string)
            n171 = VISA Write(VISA resource name=w367, write buffer=w369, error in (no error)=w366) -> (VISA resource name out=w365:refnum<visa-resource-name>, error out=w364:errorcluster)  [unwired: 1 out]
          }
          frame #13 {
            n172 = Wait (ms)(milliseconds to wait=u32 150) -> ()  [unwired: 1 out]
          }
          frame #14 {
            w382 = ":LEADing\n:TRAiling "  # Channel
            w387 = ":PULSe:TRANsition"  # VOLTage:Offset
            n173 = local read "上升下降沿"() -> (w383:i32)
            n174 = Pick Line(multi-line string=w382, line index=w383) -> (output string=w379:string)  [unwired: 1 in]
            n175 = Number To Fractional String(use system decimal point (T)=TRUE ("使用系统小数点(T)"), number="上升下降沿/s") -> (F-format string=w380:string)  [unwired: 2 in]
            n176 = Concatenate Strings(w381, w387, w379, w380) -> (w384:string)
            n177 = VISA Write(VISA resource name=w378, write buffer=w384, error in (no error)=w377) -> (VISA resource name out=w376:refnum<visa-resource-name>, error out=w375:errorcluster)  [unwired: 1 out]
          }
        }
        n178 = VISA Close(VISA resource name=w293, error in (no error)=w292) -> (error out=→"configure error out":errorcluster)
      }
    }
    n179 = event shown="[1] \"Output 1\": 值改变" {
      selector: _ -> [_ _]
      dyn-events: _ -> [_ _]
      timeout: u32 0 ("Time") -> [_ _]
      tunnel: "Output 1" -> [_ w165]
      event Timeout {
        n180 = event-data() -> ()  [unwired: 1 in, 2 out]
      }
      event "Output 1": Value Change {
        n181 = event-data() -> ()  [unwired: 1 in, 6 out]
        n182 = local read "VISA 信号发生器"() -> (w161:refnum<visa-resource-name>)
        n183 = VISA Open(VISA resource name=w161) -> (VISA resource name=w164:refnum<visa-resource-name>, error out=w167:errorcluster)  [unwired: 4 in]
        n184 = stacked-sequence {
          tunnel: w165 -> [w172 _]
          tunnel: w167 -> [w171 _]
          tunnel: w164 -> [w170 _]
          tunnel: [w169 _] -> w163
          tunnel: [w168 _] -> w162
          frame #0 {
            n185 = case shown="真" w172 {
              tunnel: w170 -> [w180 w188]
              tunnel: [w179 w187] -> w168
              tunnel: w171 -> [w178 w185]
              tunnel: [w177 w186] -> w169
              frame True {
                n186 = local write "Output"(TRUE ("布尔")) -> ()
                n187 = local read "channel输出口"() -> (w174:i32)
                n188 = Pick Line(multi-line string=":OUTP1 ON\n:OUTP2 ON" ("write buffer"), line index=w174) -> (output string=w173:string)  [unwired: 1 in]
                n189 = VISA Write(VISA resource name=w180, write buffer=w173, error in (no error)=w178) -> (VISA resource name out=w177:refnum<visa-resource-name>, error out=w179:errorcluster)  [unwired: 1 out]
              }
              frame False {
                n190 = local read "channel输出口"() -> (w182:i32)
                n191 = Pick Line(multi-line string=":OUTP1 OFF\n:OUTP2 OFF" ("write buffer"), line index=w182) -> (output string=w181:string)  [unwired: 1 in]
                n192 = VISA Write(VISA resource name=w188, write buffer=w181, error in (no error)=w185) -> (VISA resource name out=w186:refnum<visa-resource-name>, error out=w187:errorcluster)  [unwired: 1 out]
                n193 = local write "Output"(FALSE ("布尔")) -> ()
              }
            }
          }
          frame #1 {
            n194 = Wait (ms)(milliseconds to wait=u32 150) -> ()  [unwired: 1 out]
          }
        }
        n195 = VISA Close(VISA resource name=w163, error in (no error)=w162) -> (error out=→"output control error  5":errorcluster)
      }
    }
  }
  n196 = flat-sequence {
    frame #0 {
      "Backlight" <- i32[][] [] ("Backlight")
      "data 2" <- i32[][] [] ("data 2")
    }
    frame #1 {
      w390 = FALSE
      # "删除背景光控件\n初始值设定"
      n197 = local write "cut backlight"(w390) -> ()
      "backlight" <- w390
    }
  }
  n198 = stacked-sequence {
    seq-local: [_ _ _ w411 _ _ _ _] -> [_ _ _ _ w429 w449 w452 w564]
    seq-local: [_ _ _ w410 _ _ _ _] -> [_ _ _ _ w430 w450 w451 w565]
    frame #0 {
      # "initialize all variables"
      n199 = property on="initialize" class="Bool"("Désactivé"=u8 0) -> ()  [unwired: 2 in, 2 out]
      n200 = property on="Acquire" class="Bool"("Visible"=FALSE) -> ()  [unwired: 2 in, 2 out]
      n201 = property on="Setup" class="Bool"("Visible"=FALSE) -> ()  [unwired: 2 in, 2 out]
      n202 = local write "indicator"("" ("indicator")) -> ()
      n203 = local write "initialized ?"(FALSE ("initialized ?")) -> ()
      n204 = local write "Continuous"(FALSE ("Continuous")) -> ()
      n205 = local write "Close"(FALSE ("Close")) -> ()
      n206 = property on="Device Name" class="Ring (严格)"("Désactivé"=u8 0) -> ()  [unwired: 2 in, 2 out]
      n207 = property on="Continuous" class="Bool (严格)"("Visible"=FALSE) -> ()  [unwired: 2 in, 2 out]
      n208 = local write "Commande tab"(T1."Settings" ("Commande tab")) -> ()
    }
    frame #1 {
      # "Read Uniq ID"
      n209 = stacked-sequence {
        frame #0 {
          n210 = call "read detector uniq-id.vi"() -> ("nbr of components"=w403:i32, "UniqueID"=w402:string[], "Name"=w401:string[])  [unwired: 4 out]
          n211 = for {
            N: w403 -> [_]
            tunnel: w402 -> [w405]
            tunnel: w401 -> [w404]
            n212 = property on="Device Name" class="Ring (严格)"("Chaînes []"=w404) -> ()  [unwired: 2 in, 2 out]
            n213 = property on="Uniques ID" class="Ring (严格)"("Chaînes []"=w405) -> ()  [unwired: 2 in, 2 out]
          }
        }
      }
    }
    frame #2 {
      n214 = while {
        stop <- "initialize" stop-if-true
        n215 = local read "Device Name"() -> (w408:u16)
        n216 = local write "Uniques ID"(w408) -> ()
        n217 = local read "Close"() -> (w406:bool)
        n218 = Stop(stop? (T)=w406) -> ()
        n219 = Wait Until Next ms Multiple(millisecond multiple=u32 100 ("n millisecondes")) -> ()  [unwired: 1 out]
      }
    }
    frame #3 {
      n220 = stacked-sequence {
        tunnel: [_ w418 _ _] -> w411
        tunnel: [_ w417 _ _] -> w410
        frame #0 {
          n221 = local write "indicator"("Initializing ..." ("indicator")) -> ()
        }
        frame #1 {
          n222 = local read "Uniques ID"() -> (w415:u16)
          n223 = property on="Uniques ID" class="Ring (严格)"() -> ("Chaînes []"=w416:string[])  [unwired: 2 in, 2 out]
          n224 = Index Array(array=w416, index=w415) -> (element=w414:string)
          n225 = call "Initialize CCD.vi"("Unique id:"=w414) -> ("activeYPixels"=→"Y Pixels:":i32, "JYCCDLib.IJYCCDReqd"=w417:refnum<k7>, "activeXPixels"=→"X Pixels:":i32, "sortie d'erreur"=w418:errorcluster, "FirmwareVersion"=→"Firmware\nVersion":string)  [unwired: 3 out]
        }
        frame #2 {
          n226 = property on="initialize" class="Bool"("Désactivé"=u8 2) -> ()  [unwired: 2 in, 2 out]
          n227 = property on="Device Name" class="Ring (严格)"("Désactivé"=u8 2) -> ()  [unwired: 2 in, 2 out]
          n228 = local write "Continuous"(FALSE ("Continuous")) -> ()
          n229 = property on="Setup" class="Bool"("Visible"=TRUE) -> ()  [unwired: 2 in, 2 out]
        }
        frame #3 {
          n230 = local write "initialized ?"(TRUE ("initialized ?")) -> ()
          n231 = local write "indicator"("Initialized !" ("indicator")) -> ()
        }
      }
    }
    frame #4 {
      # "Actually not working"
      # "Read ADC and GAIN"
      n232 = case shown="真" "Constante de condition\n(Voir l'aide contextuelle)" {
        tunnel: w430 -> [_ w440]
        tunnel: w429 -> [_ w439]
        frame False {
        }
        frame True {
          # "Read Input supported trigger"
          n233 = call "Trigger - Get Supported Input.vi"("JYCCDLib.IJYCCDReqd"=w440, "Error Input"=w439) -> ("trigAddress"=w434:i32, "eventPtr"=w435:i32, "trigEventString"=w438:string, "trigSigType"=w437:i32, "trigSigTypeString"=w436:string)  [unwired: 4 out]
          n234 = local write "trigSigTypeString"(w436) -> ()
          n235 = local write "trigAddress"(w434) -> ()
          n236 = local write "Trigger Type :"(w435) -> ()
          n237 = local write "trigEventString"(w438) -> ()
          n238 = local write "Signal type :"(w437) -> ()
        }
      }
      n239 = call "Init ADC & Gain.vi"("JYCCDLib.IJYCCDReqd"=w430, "input error"=w429) -> ("ADC Number"=w428:i32[], "ADC description"=w433:string[], "Gain Number"=w431:i32[], "Gain description"=w432:string[])
      n240 = local write "Gain Number"(w431) -> ()
      n241 = local write "ADC Number"(w428) -> ()
      n242 = stacked-sequence {
        tunnel: w433 -> [w441 _]
        tunnel: w432 -> [_ w442]
        frame #0 {
          n243 = property on="ADC" class="Ring (严格)"("Chaînes []"=w441) -> ()  [unwired: 2 in, 2 out]
        }
        frame #1 {
          n244 = property on="GAIN" class="Ring (严格)"("Chaînes []"=w442) -> ()  [unwired: 2 in, 2 out]
        }
      }
    }
    frame #5 {
      # "IS multi Accumulation Supported ?"
      n245 = call "MultiAccu - Is Supported.vi"("Error In"=w449, "JYCCDLib.IJYCCDReqd"=w450) -> ("IsOperatingModeSupported"=w443:bool)  [unwired: 3 out]
      n246 = Select(t=0, s=w443, f=2) -> (s? t:f=w446:i32)
      n247 = Select(t=FALSE, s=w443, f=w443) -> (s? t:f=w445:bool)
      n248 = local write "Multi Accumulation mode:"(w445) -> ()
      n249 = property on="Multi Accumulation mode:" class="Bool (严格)"("Désactivé"=w446) -> ()  [unwired: 2 in, 2 out]
      n250 = property on="Multi Accumulation mode:" class="Bool (严格)"("Désactivé"=w446) -> ()  [unwired: 2 in, 2 out]
    }
    frame #6 {
      n251 = while {
        tunnel: w451 -> [w459]
        tunnel: w452 -> [w458]
        stop <- "Close" stop-if-true
        n252 = case shown="真" "Reformat" {
          frame False {
          }
          frame True {
            n253 = local read "Y Pixels:"() -> (w542:i32)
            n254 = local read "X Pixels:"() -> (w544:i32)
            n255 = call "Spectral Reformat CCD area.vi"("Y Pixels:"=w542, "X Pixels:"=w544, "numAreas"="Number of Areas :") -> ("areas :"=→"areas :":i32[][])  [unwired: 3 out]
          }
        }
        n256 = case shown="真" "Setup" {
          tunnel: w458 -> [_ w547]
          tunnel: w459 -> [_ w546]
          frame False {
          }
          frame True {
            n257 = stacked-sequence {
              tunnel: w547 -> [_ w561 _]
              tunnel: w546 -> [_ w549 _]
              frame #0 {
                n258 = local write "indicator"("Setting up the detector" ("indicator")) -> ()
              }
              frame #1 {
                w559 = 1 items=["JYMCD_ACQ_FORMAT_IMAGE", "JYMCD_ACQ_FORMAT_SCAN"] ("Acquisition type")
                n259 = local read "Gain Number"() -> (w554:i32[])
                n260 = local read "GAIN"() -> (w550:u16)
                n261 = local read "ADC Number"() -> (w555:i32[])
                n262 = local read "ADC"() -> (w551:u16)
                n263 = Index Array(array=w554, index=w550) -> (element=w552:i32)
                n264 = Index Array(array=w555, index=w551) -> (element=w553:i32)
                n265 = local read "Number of Areas :"() -> (w557:u16)
                n266 = local read "areas :"() -> (w558:i32[][])
                n267 = call "Setup CCD.vi"("numAreas"=w557, "areas :"=w558, "JYCCDLib.IJYCCDReqd"=w549, "entrée d'erreur (pas d'erreur)"=w561, "Acquisition type"=w559, "Gain"=w552, "Select ADC"=w553, "Integration time(ms)"="Integration time (ms) :") -> ("DataSize"=→"DataSize":i32)  [unwired: 1 out]
                "JYCCDLib.IJYCCDReqd" <- w549
              }
              frame #2 {
                w562 = TRUE ("Visible")
                n268 = property on="Continuous" class="Bool (严格)"("Visible"=w562) -> ()  [unwired: 2 in, 2 out]
                n269 = property on="Acquire" class="Bool"("Visible"=w562) -> ()  [unwired: 2 in, 2 out]
                n270 = local write "indicator"("Ready !" ("indicator")) -> ()
              }
            }
          }
        }
        n271 = local read "Continuous"() -> (w460:bool)
        n272 = local read "Accumulations:"() -> (w455:u16)
        n273 = Or(x="Acquire", y=w460) -> (x .or. y?=w457:bool)
        n274 = case shown="真" w457 {
          tunnel: w459 -> [_ w472]
          tunnel: w458 -> [_ w471]
          tunnel: "Enable InputTriggers :" -> [_ w470]
          tunnel: "Multi Accumulation mode:" -> [_ w469]
          tunnel: w455 -> [_ w468]
          tunnel: "MultiAcqShutterMode" -> [_ w467]
          frame False {
          }
          frame True {
            n275 = stacked-sequence {
              seq-local: [_ _ w485 _ _] -> [_ _ _ w522 _]
              tunnel: w472 -> [_ w474 w489 w521 _]
              tunnel: w471 -> [_ w475 w488 w520 _]
              tunnel: w470 -> [_ w476 _ _ _]
              tunnel: w469 -> [_ _ w487 _ _]
              tunnel: w468 -> [_ _ w486 _ _]
              tunnel: w467 -> [_ _ w484 _ _]
              frame #0 {
                n276 = local write "CCD Busy"(TRUE ("CCD Busy")) -> ()
              }
              frame #1 {
                n277 = case shown="真" w476 {
                  tunnel: w475 -> [w477 w483]
                  tunnel: w474 -> [w478 w482]
                  frame False {
                    n278 = call "Trigger - Disable.vi"("Error In"=w477, "JYCCDLib.IJYCCDReqd"=w478) -> ()  [unwired: 6 out]
                  }
                  frame True {
                    n279 = local read "Trigger Type :"() -> (w479:u16)
                    n280 = local read "Signal type :"() -> (w480:enum16{"TTL Rising Edge", "TTL Falling Edge"})
                    n281 = local read "trigAddress"() -> (w481:i32)
                    n282 = call "Trigger - Enable.vi"("Error In"=w483, "sigType"=w480, "event"=w479, "trigAddress"=w481, "JYCCDLib.IJYCCDReqd"=w482) -> ()  [unwired: 3 out]
                  }
                }
              }
              frame #2 {
                n283 = case shown="真" w487 {
                  selector: w487 -> [_ w495]
                  tunnel: w489 -> [w492 w498]
                  tunnel: w488 -> [w491 w497]
                  tunnel: w486 -> [_ w496]
                  tunnel: [u16 1 ("Accumulations:") w496] -> w485
                  tunnel: w484 -> [_ w494]
                  frame False {
                    n284 = call "MultiAccu - Disable.vi"("Error In"=w491, "JYCCDLib.IJYCCDReqd"=w492) -> ()  [unwired: 4 out]
                  }
                  frame True {
                    n285 = call "MultiAccu - Configure.vi"("JYCCDLib.IJYCCDReqd"=w498, "Cleans Before"="Number of Cleans", "Accumulations:"=w496, "MultiAcqHardwareMode"=w495, "MultiAcqShutterMode"=w494, "Error In"=w497) -> ()  [unwired: 1 in, 9 out]
                  }
                }
              }
              frame #3 {
                n286 = local read "cut backlight"() -> (w508:bool)
                n287 = local read "backlight"() -> (w507:bool)
                n288 = call "MultiAccu - Acquire spectral.vi"("error in"=w520, "Accumulations:"=w522, "ShutterOpen"="ShutterOpen", "JYCCDLib.IJYCCDReqd"=w521) -> ("Acq Time(ms)"=→"Acq Time(ms)":u32, "Array Out"=w519:i32[][][])  [unwired: 1 out]
                n289 = And(x=w508, y=w507) -> (x .and. y?=w509:bool)
                n290 = call "Array reset dimension.vi"("Area Number"="Area Number to Display", "Array In"=w519) -> ("Array Out"=w502:i32[][])
                n291 = case shown="真" w509 {
                  tunnel: [w525 w526] -> w510
                  tunnel: w502 -> [w525 w527]
                  frame False {
                  }
                  frame True {
                    n292 = local read "Backlight"() -> (w528:i32[][])
                    n293 = Subtract(x=w527, y=w528) -> (x-y=w526:i32[][])
                  }
                }
                n294 = TCP Open Connection(address="地址", remote port or service name="端口") -> (connection ID=w506:refnum<k5>)  [unwired: 3 in, 1 out]
                n295 = local write "Data"(w502) -> ()
                n296 = local write "data 2"(w502) -> ()
                n297 = local read "波长范围"() -> (w513:dbl[])
                n298 = Index Array(array=w510, index (row)=0 ("禁用的索引 (列)")) -> (element=w512:i32[])  [unwired: 1 in]
                n299 = Reverse 1D Array(array=w512) -> (reversed array=w511:i32[])
                n300 = call "转换至动态数据2"("Array"=w513) -> ("Dynamic Data Type"=w515:dynamicdata)  [unwired: 3 in]
                n301 = call "转换至动态数据"("Array"=w511) -> ("Dynamic Data Type"=w516:dynamicdata)  [unwired: 3 in]
                n302 = call "Build XY Graph2"("Y Input"=w516, "X Input"=w515) -> ("XY Graph"=w514:cluster{"Y":dbl[], "Y":dbl[]}[])  [unwired: 8 in, 1 out]
                n303 = local write "Spectrum"(w514) -> ()
                n304 = Array To Spreadsheet String(delimiter (Tab)="分隔符(Tab)", array=w502, 3:"格式字符串") -> (spreadsheet string=w501:string)
                n305 = TCP Write(connection ID=w506, data in=w501) -> (connection ID out=w505:refnum<k5>)  [unwired: 2 in, 2 out]
                n306 = TCP Close Connection(connection ID=w505) -> ()  [unwired: 2 in, 2 out]
              }
              frame #4 {
                n307 = case shown="真" "Save Backlight" {
                  frame False {
                  }
                  frame True {
                    w531 = TRUE ("删除背景光")
                    n308 = local read "Data"() -> (w533:i32[][])
                    n309 = local write "Backlight"(w533) -> ()
                    n310 = local write "cut backlight"(w531) -> ()
                    n311 = local write "backlight"(w531) -> ()
                    n312 = local write "Save Backlight"(FALSE ("Save Backlight")) -> ()
                  }
                }
                n313 = local write "CCD Busy"(FALSE ("CCD Busy")) -> ()
              }
            }
          }
        }
        n314 = case shown="真" "Temperature" {
          tunnel: w459 -> [_ w536]
          tunnel: w458 -> [_ w535]
          frame False {
            n315 = property on="temp graph" class="WFChart (严格)"("Visible"=FALSE) -> ()  [unwired: 2 in, 2 out]
          }
          frame True {
            n316 = stacked-sequence {
              tunnel: w536 -> [_ w541]
              tunnel: w535 -> [_ w540]
              frame #0 {
                n317 = property on="temp graph" class="WFChart (严格)"("Visible"=TRUE) -> ()  [unwired: 2 in, 2 out]
              }
              frame #1 {
                w539 = u16 0 items=["° Celsius", "Kelvin", "° Farenheit"] ("units")
                n318 = call "read temperature.vi"("entrée d'erreur (pas d'erreur)"=w540, "units"=w539, "JYCCDLib.IJYCCDReqd"=w541) -> ("Current Temperature"=w538:dbl)
                n319 = local write "temp graph"(w538) -> ()
              }
            }
          }
        }
        n320 = Wait Until Next ms Multiple(millisecond multiple=u32 50 ("n millisecondes")) -> ()  [unwired: 1 out]
      }
    }
    frame #7 {
      n321 = Close Reference(reference=w565, error in (no error)=w564) -> ()  [unwired: 1 out]
    }
  }
  n322 = stacked-sequence {
    seq-local: [_ _ w575 _ _] -> [_ _ _ w585 w590]
    seq-local: [_ _ w574 _ _] -> [_ _ _ w584 _]
    seq-local: [_ _ _ w583 _] -> [_ _ _ _ _]
    frame #0 {
      n323 = call "Get Monos From Config Browser.vi"() -> ("UniqueIDs"=w570:string[], "Mono ID"=w571:string[])  [unwired: 3 in, 1 out]
      n324 = Build Cluster Array(w571, w570) -> (w568:cluster{"String":string, "String":string}[])
      n325 = property on="Mono ID" class="CmbBox"("Strings And Values []"=w568) -> ()  [unwired: 2 in, 2 out]
      n326 = Index Array(array=w568, index=0) -> (element=w569:cluster{"String":string, "String":string})
      n327 = Unbundle(w569) -> ("String"=w566:string)  [unwired: 1 out]
      "Current UniqueID" <- w566
      n328 = local write "Mono ID"(w566) -> ()
    }
    frame #1 {
      n329 = while {
        stop <- "Connect" stop-if-true
        n330 = local read "Mono ID"() -> (w572:string)
        n331 = local write "Current UniqueID"(w572) -> ()
      }
    }
    frame #2 {
      n332 = local read "Mono ID"() -> (w577:string)
      n333 = call "JYInitMono.vi"("Unique ID"=w577, "Force Init"="Force\nInitialization") -> ("Refnum out"=w575:refnum<k7>, "Initialized"=→"Initialized JY":bool, "error out"=w574:errorcluster)  [unwired: 9 in, 2 out]
    }
    frame #3 {
      n334 = call "Show Current Grating.vi"("Refnum in"=w585, "error in (no error)"=w584) -> ("Gratings"=w586:dbl[], "Grating Index"=w580:i32, "Current Grating"=w582:dbl, "Current Description"=w579:string, "error out"=w583:errorcluster)  [unwired: 5 in, 4 out]
      "Gratings" <- w586
      n335 = local write "Current Grating"(w582) -> ()
      n336 = local write "Current Description"(w579) -> ()
      n337 = Number To Decimal String(number=w586) -> (decimal integer string=w588:string[])  [unwired: 1 in]
      n338 = Number To Decimal String(number=w580) -> (decimal integer string=w581:string)  [unwired: 1 in]
      n339 = property on="Target Grating" class="CmbBox"("Value"=w581) -> ()  [unwired: 2 in, 2 out]
      n340 = Build Cluster Array(w588, string[] ["1", "2", "3"]) -> (w589:cluster{"Numeric":string, string}[])
      n341 = property on="Target Grating" class="CmbBox"("Strings And Values []"=w589) -> ()  [unwired: 2 in, 2 out]
    }
    frame #4 {
      n342 = while {
        tunnel: w590 -> [w592]
        stop <- w591 stop-if-true
        n343 = stacked-sequence {
          seq-local: [w596 _ _ _ _] -> [_ w603 w614 _ w622]
          seq-local: [w595 _ _ _ _] -> [_ w602 w613 _ _]
          seq-local: [_ w601 _ _ _] -> [_ _ _ _ _]
          seq-local: [_ w600 _ _ _] -> [_ _ _ _ _]
          seq-local: [_ _ w606 _ _] -> [_ _ _ _ _]
          seq-local: [_ _ w605 _ _] -> [_ _ _ w616 _]
          tunnel: w592 -> [w594 _ _ w617 _]
          frame #0 {
            n344 = call "Show Current Grating.vi"("Refnum in"=w594) -> ("Grating Index"=→"Grating Index":i32, "Current Grating"=→"Current Grating":dbl, "Current Description"=→"Current Description":string, "error out"=w595:errorcluster, "JYMONOLib.IJYMonoReqd"=w596:refnum<k7>)  [unwired: 6 in, 4 out]
          }
          frame #1 {
            n345 = call "JYGetCurrentWL.vi"("error in (no error)"=w602, "JYMONOLib.IJYMonoReqd"=w603) -> ("error out"=w600:errorcluster, "Units"=→"Units":string, "Current WL"=→"Current WL":dbl, "JYMONOLib.IJYMonoReqd 2"=w601:refnum<k7>)  [unwired: 6 in]
          }
          frame #2 {
            w611 = u16 1 items=["Entrance", "Exit"] ("Mirror Number")
            w612 = u16 0 items=["Entrance", "Exit"] ("Mirror Number")
            n346 = call "JYGetMirrorPos.vi"("error in (no error)"=w613, "Mirror"=w612, "Refnum In"=w614) -> ("error out"=w609:errorcluster, "Current Mirror Position"=→"Entrance Mirror\nPosition":i32, "Refnum Out"=w610:refnum<k7>)  [unwired: 1 in]
            n347 = call "JYGetMirrorPos.vi"("error in (no error)"=w609, "Mirror"=w611, "Refnum In"=w610) -> ("error out"=w605:errorcluster, "Current Mirror Position"=→"Exit Mirror\nPosition":i32, "Refnum Out"=w606:refnum<k7>)  [unwired: 1 in]
          }
          frame #3 {
            w619 = u16 0 items=["Front Entrance", "Side Entrance", "Front Exit", "Side Exit", "First Intermediate", "Second Intermediate"] ("Slit")
            n348 = call "JYGetSlits.vi"("MonoRefNum IN"=w617, "Slit"=w619, "error in (no error)"=w616) -> ("Units"=→"Units 2":string, "Slit Width"=→"Front Entrance":dbl, "error out"=→"error out":errorcluster)  [unwired: 13 in, 1 out]
          }
          frame #4 {
            n349 = case shown="真" "Move To\nTarget Positions" {
              tunnel: w622 -> [_ w623]
              frame False {
              }
              frame True {
                n350 = stacked-sequence {
                  seq-local: [w625 _ _ _] -> [_ w631 _ _]
                  seq-local: [_ w629 _ _] -> [_ _ w646 _]
                  seq-local: [_ _ w633 _] -> [_ _ _ w652]
                  seq-local: [_ _ _ w649] -> [_ _ _ _]
                  tunnel: w623 -> [w627 w630 w644 w653]
                  frame #0 {
                    n351 = property on="Target Grating" class="CmbBox"() -> ("Value"=w624:string)  [unwired: 2 in, 2 out]
                    n352 = local read "error out"() -> (w626:errorcluster)
                    n353 = Decimal String To Number(string=w624) -> (number=w628:i32)  [unwired: 2 in, 1 out]
                    n354 = call "JYTurret.vi"("error in (no error)"=w626, "Grating Index"=w628, "JYMONOLib.IJYMonoReqd"=w627) -> ("error out"=w625:errorcluster)  [unwired: 2 out]
                  }
                  frame #1 {
                    # "Move Grating to Target Position"
                    n355 = call "JYMoveToWavelength.vi"("error in (no error)"=w631, "Target WL"="Target WL", "RefNum In"=w630) -> ("error out"=w629:errorcluster)  [unwired: 1 in, 2 out]
                  }
                  frame #2 {
                    w639 = u16 1 items=["Entrance", "Exit"] ("Mirror Number")
                    w638 = u16 0 items=["Entrance", "Exit"] ("Mirror Number")
                    w645 = u16 1 items=["Entrance", "Exit", "Front", "Side"] ("Mirror Number")
                    w648 = u16 0 items=["Entrance", "Exit", "Front", "Side"] ("Mirror Number")
                    # "Move Mirrors"
                    n356 = call "JYMirrorMove.vi"("error in (no error)"=w646, "Mirror Position"="Entrance Mirror", "Mirror Number"=w648, "RefNum In"=w644) -> ("error out"=w643:errorcluster)  [unwired: 6 in, 1 out]
                    n357 = call "JYMirrorMove.vi"("error in (no error)"=w643, "Mirror Position"="Exit Mirror", "Mirror Number"=w645, "RefNum In"=w644) -> ("error out"=w636:errorcluster, "MonoRefNum Out"=w637:refnum<k7>)  [unwired: 6 in]
                    n358 = call "JYGetMirrorPos.vi"("error in (no error)"=w636, "Mirror"=w638, "Refnum In"=w637) -> ("error out"=w641:errorcluster, "Current Mirror Position"=w635:i32, "Refnum Out"=w640:refnum<k7>)  [unwired: 1 in]
                    n359 = local write "Entrance Mirror\nPosition"(w635) -> ()
                    n360 = call "JYGetMirrorPos.vi"("error in (no error)"=w641, "Mirror"=w639, "Refnum In"=w640) -> ("error out"=w633:errorcluster, "Current Mirror Position"=w634:i32)  [unwired: 1 in, 1 out]
                    n361 = local write "Exit Mirror\nPosition"(w634) -> ()
                  }
                  frame #3 {
                    w651 = u16 0 items=["Front Entrance", "Side Entrance", "Front Exit", "Side Exit", "First Intermediate", "Second Intermediate"] ("Slit")
                    # "Set New Slit Positions"
                    n362 = call "JYSlits.vi"("JYMONOLib.IJYMonoReqd"=w653, "Slit"=w651, "error in (no error)"=w652, "Slit Width"="Target\nFront Entrance") -> ("error out"=w649:errorcluster)  [unwired: 1 in, 1 out]
                  }
                }
              }
            }
          }
        }
        n363 = local read "Close"() -> (w591:bool)
      }
    }
  }
  n364 = for {
    N: 1024 -> [_]
    tunnel: [w658] -> w3 mode=indexing
    i -> [w660]
    n365 = Subtract(x="终止波长", y="起始波长") -> (x-y=w656:dbl)
    n366 = Divide(x=w656, y=1024.0) -> (x/y=w654:dbl)
    n367 = Multiply(x=w654, y=w660) -> (x*y=w659:dbl)
    n368 = Add(x=w659, y="起始波长") -> (x+y=w658:dbl)
  }
  "波长范围" <- w3
